vi "Calculate Update Time.vi"(8 "error in (no error)":errorcluster, 10 "previous configuration in":refnum<class "SV Signal.lvclass">, 11 "new configuration in":refnum<class "SV Signal.lvclass">) -> (0 "error out":errorcluster, 1 "actual transition time":dbl, 2 "previous configuration out":refnum<class "SV Signal.lvclass">, 3 "new configuration out":refnum<class "SV Signal.lvclass">)   [LabVIEW 2017, in "SV Signal.lvclass"]
uses:
  <vilib>/addons/_NISVFA/_Generation/Signal Generation/SV Signal/SV Signal.lvclass
  <vilib>/addons/_NISVFA/_Generation/Signal Generation/SV Signal/SV Signal.lvclass/SV Signal.ctl
  <vilib>/addons/_NISVFA/_Generation/subVIs/sv_Optimum Location.ctl
  <vilib>/addons/_NISVFA/_Generation/SoundVib_Generation.lvlib
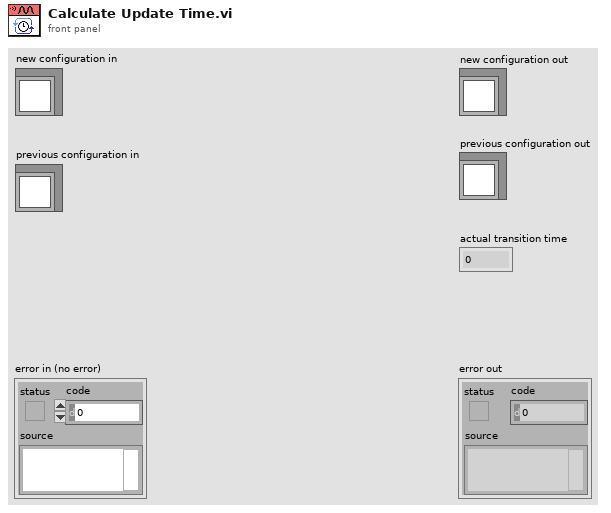
[diagram p1: front panel]
types:
  T1 = typedef "SoundVib_Generation.lvlib/sv_Optimum Location.ctl" = enum16{"Zero Crossing, First Available", "Zero Crossing, Positive Slope", "Zero Crossing, Negative Slope", "Peak or Valley", "Peak", "Valley"}
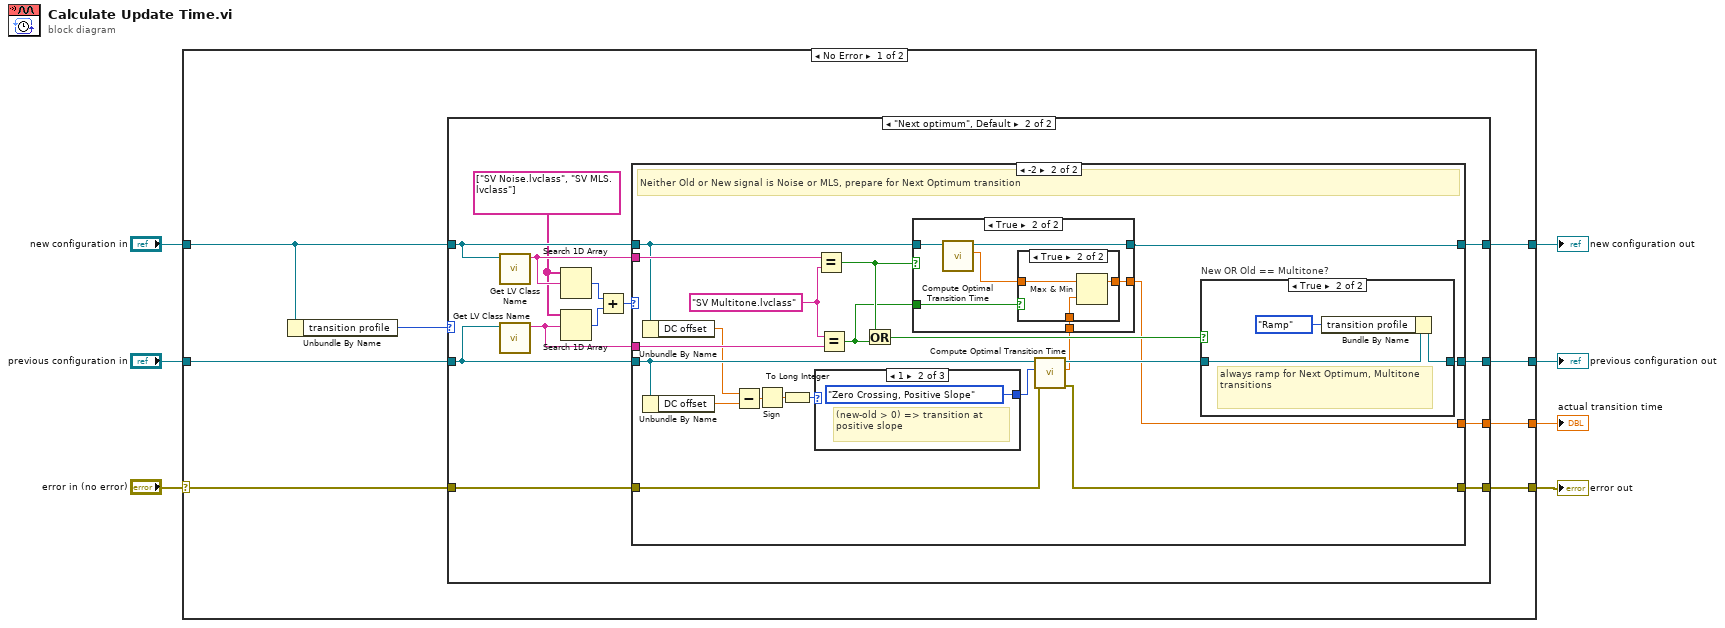
[diagram p0: block diagram]
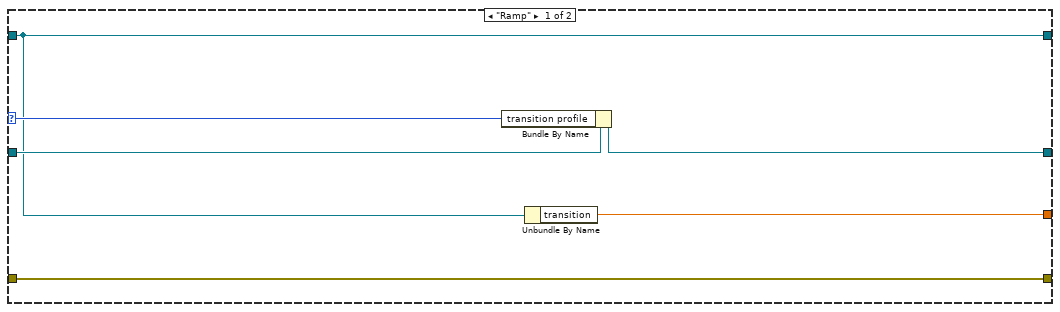
[diagram p2: hidden frame]
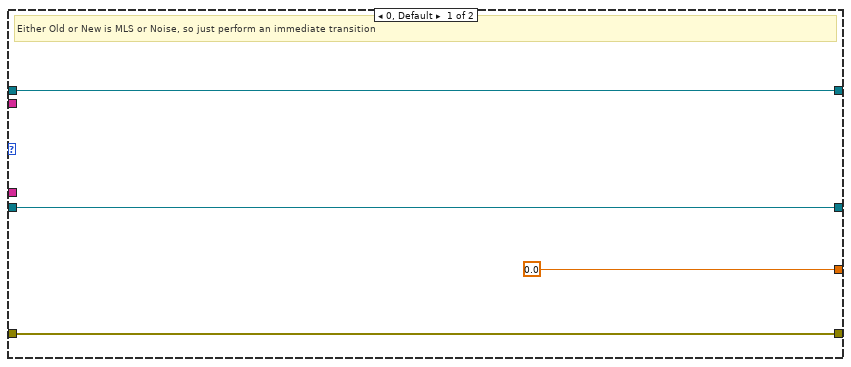
[diagram p3: hidden frame]
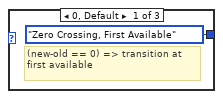
[diagram p6: hidden frame]
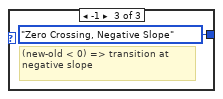
[diagram p7: hidden frame]
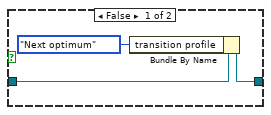
[diagram p8: hidden frame]
diagram:
  n1 = case shown="No Error" "error in (no error)" {
    selector: "error in (no error)" -> [w15 w83]
    tunnel: [w10 w83] -> w6
    tunnel: [w11 w82] -> w4
    tunnel: "new configuration in" -> [w13 w82]
    tunnel: "previous configuration in" -> [w14 w81]
    tunnel: [w9 w81] -> w2
    tunnel: [w8 _] -> w1
    frame No Error {
      n2 = Unbundle By Name(w13) -> ("transition profile"=w12:enum16{"Immediate", "Next optimum", "Ramp"})
      n3 = case shown="\"Next optimum\", Default" w12 {
        selector: w12 -> [w19 _]
        tunnel: [w18 w34] -> w11
        tunnel: w13 -> [w18 w30]
        tunnel: w14 -> [w21 w29]
        tunnel: [w20 w33] -> w9
        tunnel: w15 -> [w17 w31]
        tunnel: [w17 w32] -> w10
        tunnel: [w16 w22] -> w8
        frame "Ramp" {
          n4 = Bundle By Name(cluster=w21, "transition profile"=w19) -> (w20:refnum<class "SV Signal.lvclass">)
          n5 = Unbundle By Name(w18) -> ("transition"=w16:dbl)
        }
        frame "Next optimum", Default {
          w26 = string[] ["SV Noise.lvclass", "SV MLS.lvclass"] ("1D array")
          n6 = call <vilib>:"Get LV Class Name.vi"("object"=w30) -> ("class name"=w28:string)  [unwired: 9 in, 1 out]
          n7 = call <vilib>:"Get LV Class Name.vi"("object"=w29) -> ("class name"=w27:string)  [unwired: 9 in, 1 out]
          n8 = Search 1D Array(1D array=w26, element=w28) -> (index of element=w25:i32)  [unwired: 1 in]
          n9 = Search 1D Array(1D array=w26, element=w27) -> (index of element=w24:i32)  [unwired: 1 in]
          n10 = Add(x=w25, y=w24) -> (x+y=w23:i32)
          n11 = case shown="-2" w23 {
            tunnel: [w37 w41] -> w34
            tunnel: [w38 w59] -> w33
            tunnel: [w36 w40] -> w32
            tunnel: w31 -> [w36 w53]
            tunnel: w30 -> [w37 w45]
            tunnel: w29 -> [w38 w52]
            tunnel: w28 -> [_ w55]
            tunnel: w27 -> [_ w54]
            tunnel: [0.0 ("actual transition time") w39] -> w22
            frame 0, Default {
              # "Either Old or New is MLS or Noise, so just perform an immediate transition"
            }
            frame -2 {
              w58 = "SV Multitone.lvclass" ("y")
              # "Neither Old or New signal is Noise or MLS, prepare for Next Optimum transition"
              n12 = Unbundle By Name(w45) -> ("DC offset"=w51:dbl)
              n13 = Unbundle By Name(w52) -> ("DC offset"=w50:dbl)
              n14 = Subtract(x=w51, y=w50) -> (x-y=w48:dbl)
              n15 = Sign(1:w48) -> (0:w46:dbl)
              n16 = To Long Integer(number=w46) -> (32bit integer=w47:i32)
              n17 = case shown="1" w47 {
                tunnel: [sv_Optimum_Location."Zero Crossing, First Available" ("optimum") sv_Optimum_Location."Zero Crossing, Positive Slope" ("optimum") sv_Optimum_Location."Zero Crossing, Negative Slope" ("optimum")] -> w49
                frame 0, Default {
                  # "(new-old == 0) => transition at first available"
                }
                frame 1 {
                  # "(new-old > 0) => transition at positive slope"
                }
                frame -1 {
                  # "(new-old < 0) => transition at negative slope"
                }
              }
              n18 = Equal?(x=w55, y=w58) -> (x = y?=w44:bool)
              n19 = Equal?(x=w58, y=w54) -> (x = y?=w42:bool)
              n20 = Or(x=w44, y=w42) -> (x .or. y?=w57:bool)
              n21 = call-dynamic "Compute Optimal Transition Time.vi"("error in (no error)"=w53, "optimum"=w49, "SV Signal in"=w52) -> ("error out"=w40:errorcluster, "optimal transition time"=w43:dbl, "SV Signal out"=w56:refnum<class "SV Signal.lvclass">)  [unwired: 6 in]
              n22 = case shown="True" w44 {
                tunnel: w45 -> [w61 w67]
                tunnel: [w61 w66] -> w41
                tunnel: w43 -> [w60 w64]
                tunnel: w42 -> [_ w65]
                tunnel: [w60 w62] -> w39
                frame False {
                }
                frame True {
                  n23 = call-dynamic "Compute Optimal Transition Time.vi"("SV Signal in"=w67) -> ("optimal transition time"=w63:dbl, "SV Signal out"=w66:refnum<class "SV Signal.lvclass">)  [unwired: 8 in, 1 out]
                  n24 = case shown="True" w65 {
                    tunnel: w64 -> [_ w71]
                    tunnel: w63 -> [w68 w70]
                    tunnel: [w68 w69] -> w62
                    frame False {
                    }
                    frame True {
                      n25 = Max & Min(x=w70, y=w71) -> (max(x,y)=w69:dbl)  [unwired: 1 out]
                    }
                  }
                }
              }
              n26 = case "New OR Old == Multitone?" shown="True" w57 {
                tunnel: [w76 w80] -> w59
                tunnel: w56 -> [w77 w79]
                frame False {
                  n27 = Bundle By Name(cluster=w77, "transition profile"=enum16{"Immediate", "Next optimum", "Ramp"}."Next optimum") -> (w76:refnum<class "SV Signal.lvclass">)
                }
                frame True {
                  # "always ramp for Next Optimum, Multitone transitions"
                  n28 = Bundle By Name(cluster=w79, "transition profile"=enum16{"Immediate", "Next optimum", "Ramp"}."Ramp") -> (w80:refnum<class "SV Signal.lvclass">)
                }
              }
            }
          }
        }
      }
    }
    frame Error {
    }
  }
  "error out" <- w6
  "new configuration out" <- w4
  "previous configuration out" <- w2
  "actual transition time" <- w1
